vi "Target_super_simple.vi"() -> ()   [LabVIEW 2019]
uses:
  <vilib>/Platform/TimedLoop/XDataNode/timing_clust.ctl
  <vilib>/Platform/TimedLoop/XDataNode/nitl_modes.ctl
  <vilib>/Platform/TimedLoop/XDataNode/wakeup.ctl
  <vilib>/rvi/DataTransferAndStorage/Container/Common/niFpgaContainerExecOnDevCompGetState.vi
  <vilib>/rvi/Emulation/niFpgaEmulationIsFPGAContextNoSignature.vi
  <vilib>/rvi/Emulation/niFpgaSctlEmulationGetInTimedLoop.vi
  <vilib>/rvi/errors/niFpgaSetErrorForExecOnDevCompSimple.vi
  <vilib>/rvi/eio/common/nirviEmuReportErrorAndStop.vi
  <vilib>/rvi/DataTransferAndStorage/Container/Common/niFpgaContainerGetUniqueNameForEmu.vi
  <vilib>/rvi/FIFO/Fifo_Resource/nirvififoEmulationSetSize.vi
  <vilib>/rvi/FIFO/Fifo_Resource/nirviFifoEmulationQueueMgr.vi
  <instcachedir>/0/nirviFifoEmulationQueueMgr_E5CAEC123FF24DC58D834DCA3CDAA9B5.lvgen/nirviFifoEmulationQueueMgr_E5CAEC123FF24DC58D834DCA3CDAA9B5_005.vi
  <vilib>/rvi/FIFO/Fifo_Resource/nirvififoEmulationDetermineInputValidOut.vi
  <vilib>/rvi/FIFO/Fifo_Resource/nirvififoEmulationCreateLock.vi
  <vilib>/rvi/Emulation/niFpgaProcessEmulError.vi
  <vilib>/rvi/FIFO/Fifo_Resource/nirvififoEmulationObtainLock.vi
  <vilib>/rvi/FIFO/Fifo_Resource/nirvififoEmulationReleaseLock.vi
  <vilib>/rvi/occurrence/nirviWaitOnOccurrenceBase.vi
  <vilib>/rvi/errors/nirviReportUnexpectedCaseInternalError.vi
  <vilib>/rvi/errors/nirviReportUnexpectedCaseInternalError (U32).vi
  <vilib>/Utility/error.llb/Clear Errors.vi
  <vilib>/rvi/interface/RandomDataEmulation/niFpgaRandomDataHandleErrors.vi
  <vilib>/rvi/Emulation/niFpgaEmulationReportErrorSimple.vi
  <vilib>/rvi/Emulation/niFpgaGetClockAttributes.vi
  <vilib>/rvi/Emulation/niFpgaCriticalErrorInLSC.vi
  <userlib>/_NI FLP Library/FPGA/insideSCTL/FlpLib Square Root SCTL Latency 5.vi
  <vilib>/rvi/DataTransferAndStorage/Container/XNode/niFpgaContainer.xnode
  <vilib>/rvi/FIFO/Fifo_Resource/niFpgaFifoEmulationRefIn.vi
  <vilib>/platform/TimedLoop/XDataNode/XDataNode.xnode
  <vilib>/Platform/TimedLoop/XDataNode/XDNodeRunTimeDep.lvlib
panel:
  out "T4 us":u16 caption="Tick Count(Ticks)"
  out "T2 us":u16 caption="Tick Count(mSec)"
  out "T3 us":u16 caption="Tick Count(mSec)"
  out "T5 us":u16 caption="crap"
  out "T5 ticks":u32 caption="Tick Count(mSec)"
  out "T4 tick":u32 caption="Tick Count(mSec)"
  out "T3 tick":u32 caption="Tick Count(mSec)"
  out "T2 tick":u32 caption="Tick Count(mSec)"
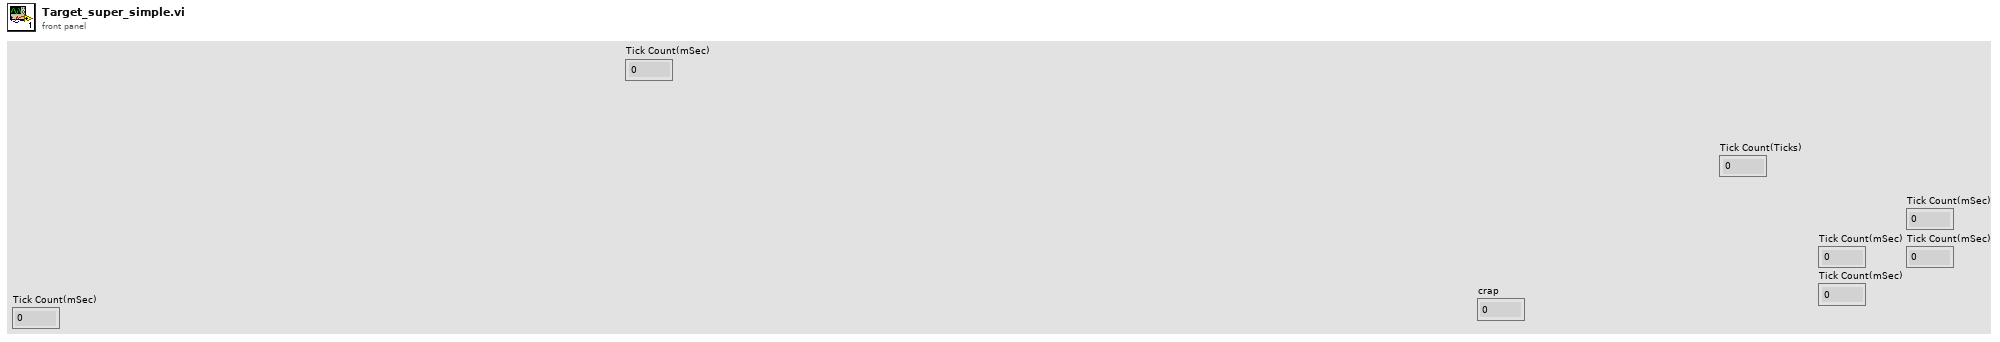
[diagram p1: front panel]
types:
  T1 = typedef "XDNodeRunTimeDep.lvlib/timing_clust.ctl" = cluster{"Expected End [f-1]":u64, "Actual End [f-1]":u64, "Finished Late? [f-1]":bool, "Expected End [i-1]":u64, "Actual End [i-1]":u64, "Finished Late? [i-1]":bool, "Expected Start [i]":u64, "Actual Start [i]":u64, "Expected Start [f]":u64, "Actual Start [f]":u64, "Source Name":string, "Structure Name":string, "Period":i64, "Deadline":i64, "Offset":i64, "Start":i64, "Priority":i32, "Timeout":i32, "Mode":T2, "Wakeup Reason":T3, "Error":errorcluster, "Source Type":string, "Secondary Source Type":string, "Global End Time":u64, "Global Start Time":u64, "Frame Duration":u64, "Iteration Duration":u64, "Assigned CPU":i32, "I/O Scan Engine Mode":u32}
  T2 = typedef "XDNodeRunTimeDep.lvlib/nitl_modes.ctl" = enum32{"No Change", "Process missed periods, maintain original phase", "Discard missed periods, maintain original phase", "Process missed periods, ignore original phase", "Discard missed periods, ignore original phase"}
  T3 = typedef "XDNodeRunTimeDep.lvlib/wakeup.ctl" = enum32{"Normal", "Aborted", "Asynchronous wakeup", "Timing source error", "Timed loop error", "Timeout"}
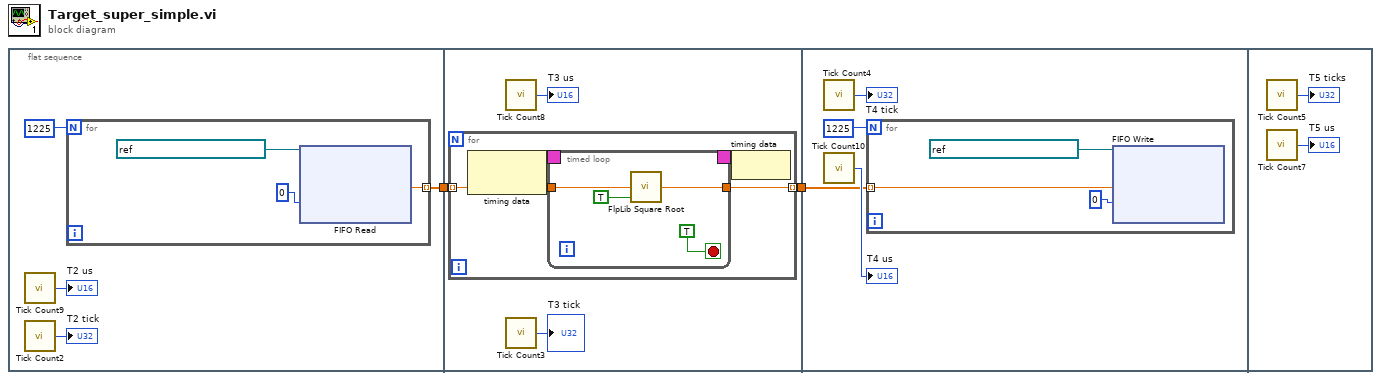
[diagram p0: block diagram]
diagram:
  n1 = flat-sequence {
    tunnel: [w3] -> w2
    tunnel: w2 -> [w11]
    tunnel: [w10] -> w1
    tunnel: w1 -> [w26]
    frame #0 {
      n2 = call "Tick Count9"() -> ("Tick Count(uSec)"=→"T2 us":u16)
      n3 = call "Tick Count2"() -> ("Tick Count(Ticks)"=→"T2 tick":u32)
      n4 = for {
        N: 1225 -> [_]
        tunnel: [w7] -> w3 mode=indexing
        n5 = xnode ("FIFO Read")("Timeout"=0, "FIFO In"=refnum<k21> "FIFO-host-to-Cholesky") -> ("Element"=w7:sgl)  [unwired: 2 out]
      }
    }
    frame #1 {
      n6 = for {
        tunnel: w11 -> [w17] mode=indexing
        tunnel: [w16] -> w10 mode=indexing
        n7 = node-c288() -> (w15:T1)  [unwired: 1 in]
        n8 = timed-loop {
          tunnel: w17 -> [w20]
          tunnel: [w19] -> w16
          timing: w15 -> [_]
          timing-out: [_] -> w14
          stop <- TRUE stop-if-true
          n9 = call-poly <userlib>:"FlpLib Square Root.vi"("input valid"=TRUE, "x"=w20) -> ("sqrt(x)"=w19:sgl)  [unwired: 2 in, 1 out]
        }
        n10 = node-c288(w14) -> ()
      }
      n11 = call "Tick Count8"() -> ("Tick Count(uSec)"=→"T3 us":u16)
      n12 = call "Tick Count3"() -> ("Tick Count(Ticks)"=→"T3 tick":u32)
    }
    frame #2 {
      n13 = call "Tick Count4"() -> ("Tick Count(Ticks)"=→"T4 tick":u32)
      n14 = call "Tick Count10"() -> ("Tick Count(uSec)"=→"T4 us":u16)
      n15 = for {
        N: 1225 -> [_]
        tunnel: w26 -> [w30] mode=indexing
        n16 = xnode ("FIFO Write")("Element"=w30, "Timeout"=0, "FIFO In"=refnum<k21> "FIFO-Cholesky-to-host") -> ()  [unwired: 2 out]
      }
    }
    frame #3 {
      n17 = call "Tick Count5"() -> ("Tick Count(Ticks)"=→"T5 ticks":u32)
      n18 = call "Tick Count7"() -> ("Tick Count(uSec)"=→"T5 us":u16)
    }
  }
